vi "sample create 150 topics.vi"() -> ()   [LabVIEW 2015]
uses:
  Topic/Topic.lvclass
  Core/HTTP Request/AWS Credentials.ctl
  Core/HTTP Request/Region.ctl
  Core/HTTP Request/HTTP Request.lvclass
panel:
  out "error out":errorcluster
  out "Topics out":refnum<class "Topic.lvclass">[](array[class])
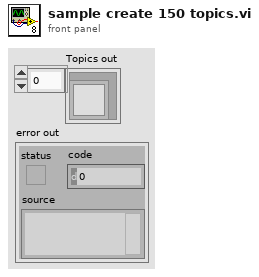
[diagram p1: front panel]
types:
  T1 = typedef "NI_AWS_Core.lvlib/HTTP Request.lvclass/Region.ctl" = enum16{"us-east-1", "us-east-2", "us-west-1", "us-west-2", "ap-northeast-1", "ap-northeast-2", "ap-southeast-1", "ap-southeast-2", "ca-central-1", "eu-central-1", "eu-west-1", "eu-west-2", "sa-east-1"}
  T2 = typedef "NI_AWS_Core.lvlib/HTTP Request.lvclass/AWS Credentials.ctl" = cluster{"Access Key":string, "Secret Key":string}
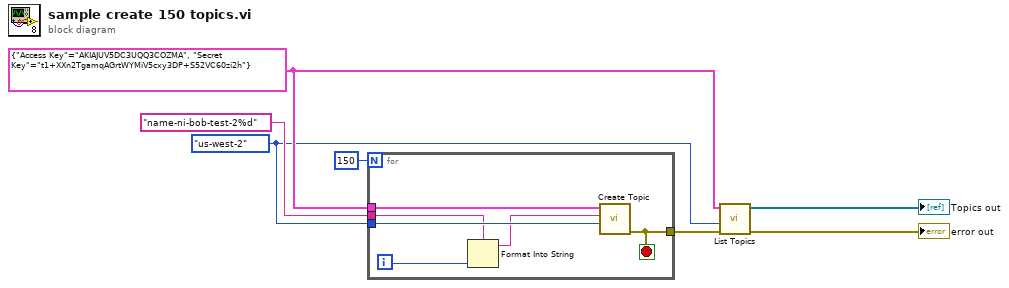
[diagram p0: block diagram]
diagram:
  w2 = Region."us-west-2" ("Region")
  w7 = T2 {"Access Key"="AKIAJUV5DC3UQQ3COZMA", "Secret Key"="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"} ("AWS Credentials")
  n1 = for {
    N: 150 -> [_]
    tunnel: w7 -> [w13]
    tunnel: "name-ni-bob-test-2%d" ("Name") -> [w10]
    tunnel: [w11] -> w4
    tunnel: w2 -> [w12]
    i -> [w8]
    stop <- w11 stop-if-true
    n2 = Format Into String(format string=w10, w8) -> (resulting string=w9:string)  [unwired: 2 in, 1 out]
    n3 = call "Create Topic.vi"("Region"=w12, "Name"=w9, "AWS Credentials"=w13) -> ("error out"=w11:errorcluster)  [unwired: 7 in, 1 out]
  }
  n4 = call "List Topics.vi"("error in (no error)"=w4, "Region"=w2, "AWS Credentials"=w7) -> ("error out"=→"error out":errorcluster, "Topics out"=→"Topics out":refnum<class "Topic.lvclass">[])  [unwired: 7 in]
